vi "Read.vi"(8 "error in (no error)":errorcluster, 11 "PVConnection in":refnum<class "PVConnection.lvclass">) -> (0 "error out":errorcluster, 2 "PV":refnum<class "PV.lvclass">, 3 "PVConnection out":refnum<class "PVConnection.lvclass">)   [LabVIEW 2013, in "CS++ProcessVariables.lvlib" / "PVConnection.lvclass"]
doc: "Read a process varibale."
uses:
  PVConnection.lvclass
  ProcessVariable/PV.lvclass
  PVConnection.lvclass/PVConnection.ctl
  ProcessVariable/PV.lvclass/PV.ctl
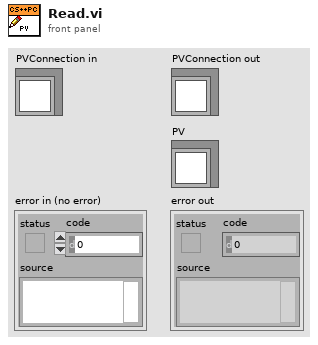
[diagram p1: front panel]
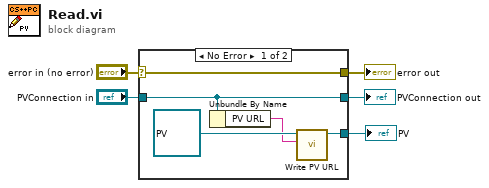
[diagram p0: block diagram]
diagram:
  n1 = case shown="No Error" "error in (no error)" {
    selector: "error in (no error)" -> [w10 w12]
    tunnel: [w10 w12] -> w4
    tunnel: [w8 w11] -> w2
    tunnel: "PVConnection in" -> [w8 w11]
    tunnel: [w6 _] -> w1
    frame No Error {
      n2 = Unbundle By Name(w8) -> ("PV URL"=w7:string)
      n3 = call "Write PV URL.vi"("PV URL"=w7, "PV in"=refnum<class "PV.lvclass"> refnum ("CS++ProcessVariables.lvlib:PV.lvclass")) -> ("PV out"=w6:refnum<class "PV.lvclass">)  [unwired: 8 in, 1 out]
    }
    frame Error {
    }
  }
  "error out" <- w4
  "PVConnection out" <- w2
  "PV" <- w1
